vi "Get MetaData from Configurations.vi"(8 "error in":errorcluster, 10 "MeasurementPluginService in":refnum<class "MeasurementPluginService.lvclass">, 11 "Configuration Cluster":variant) -> (0 "error out":errorcluster, 2 "MeasurementPluginService out":refnum<class "MeasurementPluginService.lvclass">, 3 "configuration_parameters":T1[](array[typedef]))   [LabVIEW 2020, in "MeasurementLink Measurement Server.lvlib"]
uses:
  MeasurementLink Measurement Server.lvlib
  TypeDefs/ConfigurationParameter.ctl
  TypeDefs/Parameter_AnnotationsEntry.ctl
  Classes/MeasurementPluginService/MeasurementPluginService.lvclass
  <vilib>/Utility/Data Type/NI_Data Type.lvlib
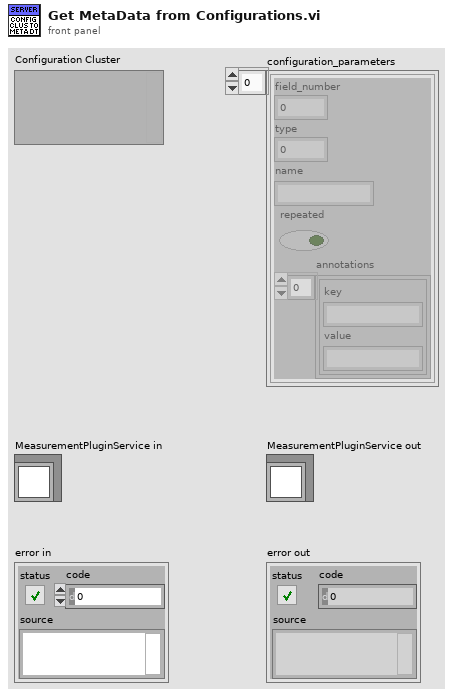
[diagram p1: front panel]
types:
  T1 = typedef "MeasurementLink Measurement Server.lvlib/ConfigurationParameter.ctl" = cluster{"field_number":i32, "type":i32, "name":string, "repeated":bool, "annotations":T2[]}
  T2 = typedef "MeasurementLink Measurement Server.lvlib/Parameter_AnnotationsEntry.ctl" = cluster{"key":string, "value":string}
  T3 = typedef "MeasurementLink Measurement Server.lvlib/MeasurementPluginService.lvclass/Plugin Paths.ctl" = cluster{"Get Measurement Details VI Path":path, "Get Type Specializations VI Path":path, "Get UI Details VI Path":path, "Measurement Logic VI Path":path, "Measurement Configuration CTL Path":path, "Measurement Results CTL Path":path}
  T4 = cluster{"Parameter Name":string, "Annotations":T2[]}[]
  T5 = typedef "NI_Data Type.lvlib/Data Type.ctl" = enum8{"Invalid Type", "Void", "I8", "I16", "I32", "I64", "U8", "U16", "U32", "U64", "Single Float", "Double Float", "Extended Float", "Single Complex", "Double Complex", "Extended Complex", "Enum U8", "Enum U16", "Enum U32", "Enum U64", "Single Float With Unit", "Double Float With Unit", "Extended Float With Unit", "Single Complex with Unit", "Double Complex with Unit", "Extended Complex with Unit", "Boolean", "String", "Path", "Picture", "Tag", "Array", "Cluster", "Variant", "LV Variant", "Waveform", "Timestamp", "Digital Waveform", "Digital Data", "ExpressData", "Refnum", "External Data", "VI", "Poly VI", "LabVIEW Class Instance", "Fixed Point", "Set Collection", "Map Collection"}
  T6 = typedef "MeasurementLink Measurement Server.lvlib/google_protobuf_Field_Kind.ctl" = enum32{"TYPE_UNKNOWN", "TYPE_DOUBLE", "TYPE_FLOAT", "TYPE_INT64", "TYPE_UINT64", "TYPE_INT32", "TYPE_FIXED64", "TYPE_FIXED32", "TYPE_BOOL", "TYPE_STRING", "TYPE_GROUP", "TYPE_MESSAGE", "TYPE_BYTES", "TYPE_UINT32", "TYPE_ENUM", "TYPE_SFIXED32", "TYPE_SFIXED64", "TYPE_SINT32", "TYPE_SINT64"}
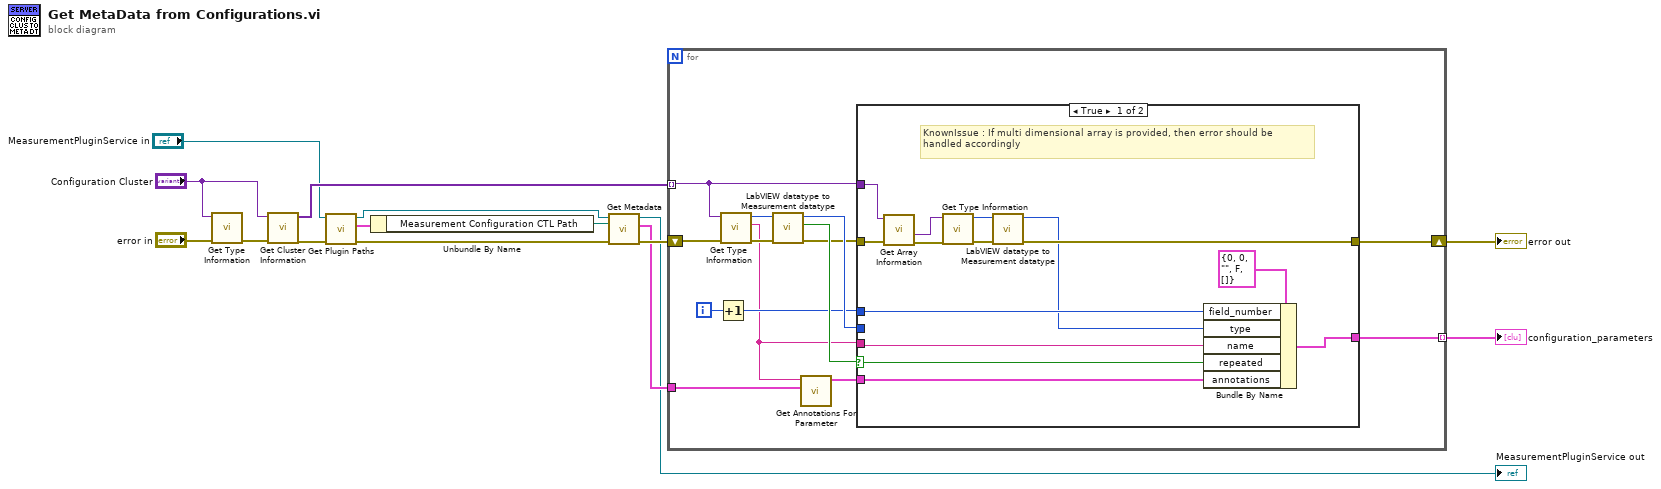
[diagram p0: block diagram]
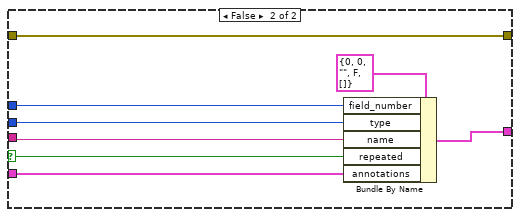
[diagram p2: hidden frame]
diagram:
  n1 = call <vilib>:"Get Type Information.vi"("error in (no error)"="error in", "variant"="Configuration Cluster") -> ("error out"=w15:errorcluster)  [unwired: 5 in, 4 out]
  n2 = call <vilib>:"Get Cluster Information.vi"("error in (no error)"=w15, "variant"="Configuration Cluster") -> ("error out"=w5:errorcluster, "cluster elements"=w14:variant[])  [unwired: 8 in]
  n3 = call-dynamic "Get Plugin Paths.vi"("error in (no error)"=w5, "MeasurementPluginService in"="MeasurementPluginService in") -> ("error out"=w8:errorcluster, "Plugin Paths"=w9:T3, "MeasurementPluginService out"=w7:refnum<class "MeasurementPluginService.lvclass">)  [unwired: 7 in]
  n4 = Unbundle By Name(w9) -> ("Measurement Configuration CTL Path"=w10:path)
  n5 = call "Get Metadata.vi"("error in (no error)"=w8, "measurement control path"=w10, "MeasurementPluginService in"=w7) -> ("error out"=w6:errorcluster, "Metadata Value"=w3:T4, "MeasurementPluginService out"=→"MeasurementPluginService out":refnum<class "MeasurementPluginService.lvclass">)  [unwired: 5 in]
  n6 = for {
    tunnel: w14 -> [w23] mode=indexing
    tunnel: [w24] -> w13 mode=indexing
    shift-right: [w19] -> w1
    shift-left: w6 -> [w29]
    tunnel: w3 -> [w16]
    i -> [w28]
    n7 = Increment(x=w28) -> (x+1=w20:i32)
    n8 = call <vilib>:"Get Type Information.vi"("error in (no error)"=w29, "variant"=w23) -> ("error out"=w22:errorcluster, "name"=w17:string, "type"=w27:T5)  [unwired: 5 in, 2 out]
    n9 = call "LabVIEW datatype to Measurement datatype.vi"("error in"=w22, "type"=w27) -> ("error out"=w21:errorcluster, "Array?"=w25:bool, "MessageElementType"=w26:T6)  [unwired: 6 in, 1 out]
    n10 = call "Get Annotations For Parameter.vi"("Metadata Value"=w16, "Parameter Name"=w17) -> ("Annotations"=w18:T2[])  [unwired: 9 in]
    n11 = case shown="True" w25 {
      selector: w25 -> [w43 w51]
      tunnel: w20 -> [w33 w47]
      tunnel: w26 -> [_ w45]
      tunnel: [w42 w50] -> w24
      tunnel: w21 -> [w41 w49]
      tunnel: w23 -> [w40 _]
      tunnel: [w36 w49] -> w19
      tunnel: w17 -> [w31 w46]
      tunnel: w18 -> [w30 w44]
      frame True {
        # "KnownIssue : If multi dimensional array is provided, then error should be handled accordingly"
        n12 = call <vilib>:"Get Array Information.vi"("error in (no error)"=w41, "variant"=w40) -> ("error out"=w39:errorcluster, "array element data type"=w35:variant)  [unwired: 6 in, 2 out]
        n13 = call <vilib>:"Get Type Information.vi"("error in (no error)"=w39, "variant"=w35) -> ("error out"=w37:errorcluster, "type"=w38:T5)  [unwired: 5 in, 3 out]
        n14 = call "LabVIEW datatype to Measurement datatype.vi"("error in"=w37, "type"=w38) -> ("error out"=w36:errorcluster, "MessageElementType"=w32:T6)  [unwired: 6 in, 2 out]
        n15 = Bundle By Name(cluster=T1 {"field_number"=0, "type"=0, "name"="", "repeated"=FALSE, "annotations"=[]} ("ConfigurationParameter"), "field_number"=w33, "type"=w32, "name"=w31, "repeated"=w43, "annotations"=w30) -> (w42:T1)
      }
      frame False {
        n16 = Bundle By Name(cluster=T1 {"field_number"=0, "type"=0, "name"="", "repeated"=FALSE, "annotations"=[]} ("ConfigurationParameter"), "field_number"=w47, "type"=w45, "name"=w46, "repeated"=w51, "annotations"=w44) -> (w50:T1)
      }
    }
  }
  "error out" <- w1
  "configuration_parameters" <- w13
